vi "Setup UI.vi"(8 "error in (no error)":errorcluster, 10 "Set UI to input? (F)":bool, 11 "Two Lockins in":refnum<class "Two Lockins.lvclass">) -> (0 "error out":errorcluster, 3 "Two Lockins out":refnum<class "Two Lockins.lvclass">)   [LabVIEW 2023, in "Two Lockins.lvclass"]
doc: "Setup UI constructs an object -- populates its member fields -- from a front panel the user can see. The VI should be as simple as possible so that a UI loop can poll it continuously for updates. \n\nThe VI is designed to be used as a subPanel within another VI. Wire true to \"Set UI to input\" only on the first call, just after inserting this VI into a subPanel, to populate its controls with the class's current values.\n\nSetup UI is distinct from the class constructor. Class constructors are not polymorphic, yet configure dialogs need to configure objects without knowing their type -- and polymorphism is the necessary solution. Thus, Setup UI is a polymorphic class constructor. This continously polled \"Setup UI\" concept is a kludge: a better idea would be an XControl, but those require a steeper learning curve."
uses:
  Two Lockins.lvclass
  Lockin/Sensitivity.ctl
  Two Lockins.lvclass/Two Lockins.ctl
  Utility Classes/Readable/Readable.lvclass
  Lockin/sr830/SR830.lvlib
  Lockin/Lockin SR830.lvclass
panel:
  in  "Tau 2":u16(ring) items=["10 us", "30 us", "100 us", "300 us", "1 ms", "3 ms", "10 ms", "30 ms", "100 ms", "300 ms", "1 s", "3 s", "10 s", "30 s", "100 s", "300 s", "1 ks", "3 ks", "10 ks", "30 ks"]
  in  "Sensitivity 2":T1 items=["2 nV", "5 nV", "10 nV", "20 nV", "50 nV", "100 nV", "200 nV", "500 nV", "1 uV", "2 uV", "5 uV", "10 uV", "20 uV", "50 uV", "100 uV", "200 uV", "500 uV", "1 mV", "2 mV", "5 mV", "10 mV", "20 mV", "50 mV", "100 mV", "200 mV", "500 mV", "1 V"]
  in  "Reference mode 2":enum16{"external", "internal"}(ring)
  in  "Frequency 2":dbl[unit]
  in  "Set Parameters":bool
  in  "Tau":u16(ring) items=["10 us", "30 us", "100 us", "300 us", "1 ms", "3 ms", "10 ms", "30 ms", "100 ms", "300 ms", "1 s", "3 s", "10 s", "30 s", "100 s", "300 s", "1 ks", "3 ks", "10 ks", "30 ks"]
  in  "Sensitivity":T1 items=["2 nV", "5 nV", "10 nV", "20 nV", "50 nV", "100 nV", "200 nV", "500 nV", "1 uV", "2 uV", "5 uV", "10 uV", "20 uV", "50 uV", "100 uV", "200 uV", "500 uV", "1 mV", "2 mV", "5 mV", "10 mV", "20 mV", "50 mV", "100 mV", "200 mV", "500 mV", "1 V"]
  in  "Reference mode":enum16{"external", "internal"}(ring)
  in  "Frequency":dbl[unit]
  # "Two Lockins Instrument Setup"
  # "SR830"
  # "SR810"
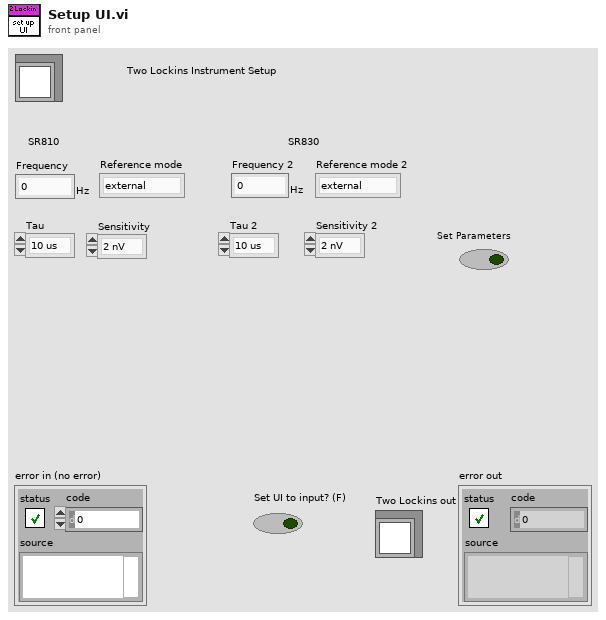
[diagram p1: front panel]
types:
  T1 = typedef "Lockin SR830.lvclass/Sensitivity.ctl" = u16
  T2 = typedef "SR830.lvlib/Tau.ctl" = u16
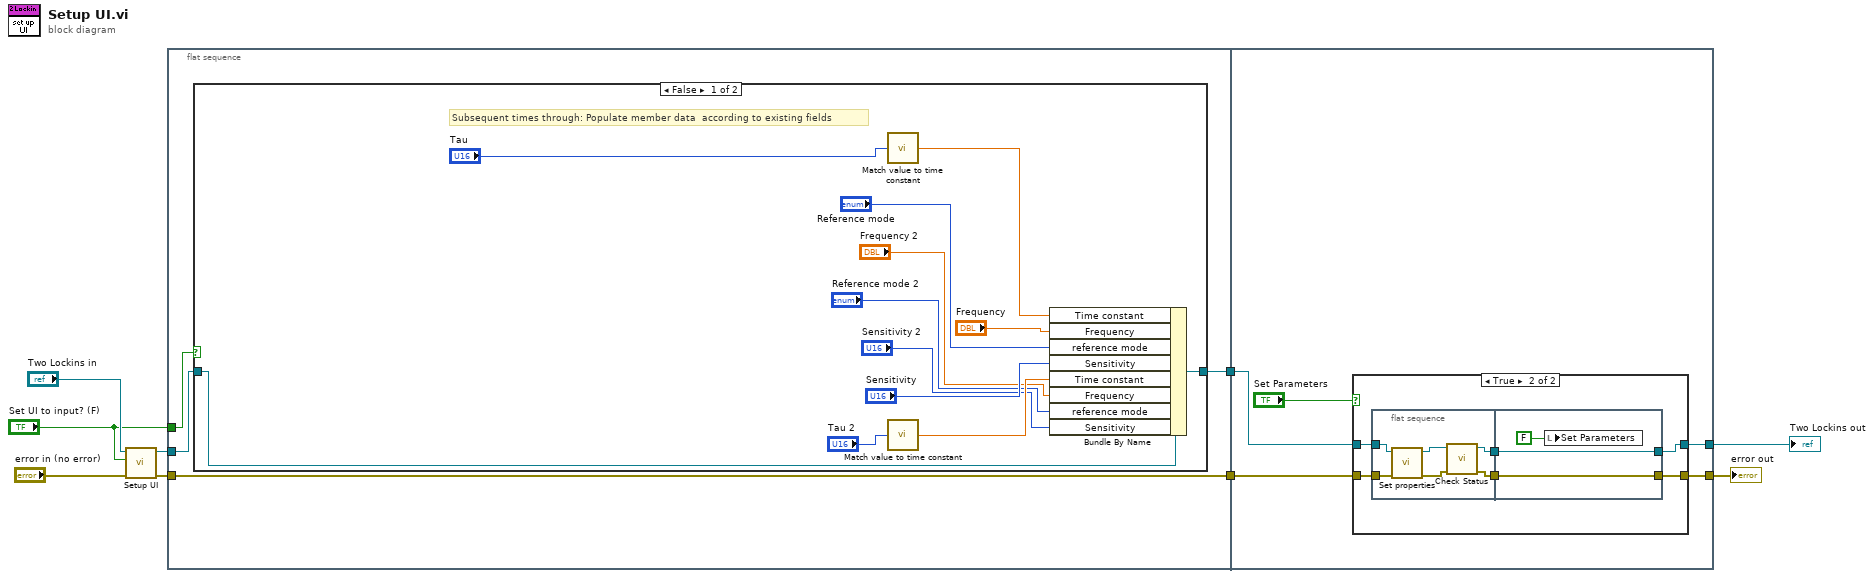
[diagram p0: block diagram]
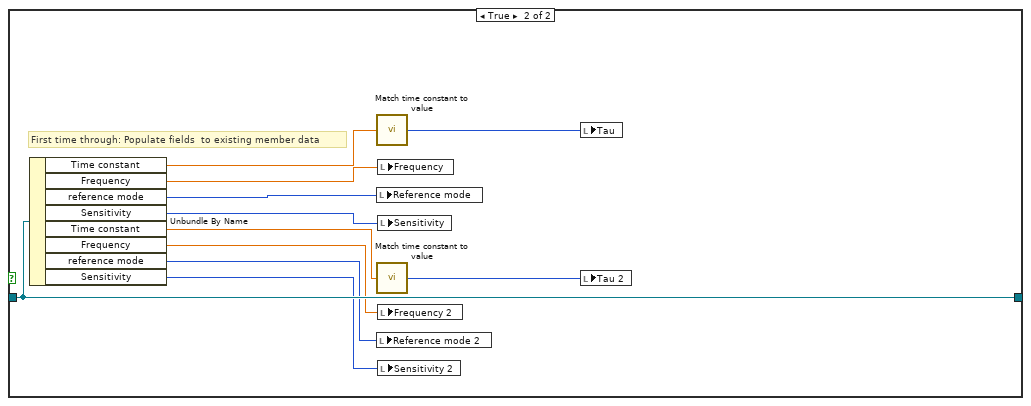
[diagram p2: hidden frame]
diagram:
  n1 = call-parent "Setup UI.vi"("error in (no error)"="error in (no error)", "Set UI to input? (F)"="Set UI to input? (F)", "Instrument in"="Two Lockins in") -> ("error out"=w4:errorcluster, "Instrument out"=w3:refnum<class "Two Lockins.lvclass">)  [unwired: 7 in]
  n2 = flat-sequence {
    tunnel: "Set UI to input? (F)" -> [w13]
    tunnel: w3 -> [w12]
    tunnel: [w11] -> w7
    tunnel: [w10] -> w6
    tunnel: w4 -> [w10]
    tunnel: w7 -> [w41]
    tunnel: [w38] -> w2
    tunnel: w6 -> [w40]
    tunnel: [w39] -> w1
    frame #0 {
      n3 = case shown="False" w13 {
        tunnel: w12 -> [w25 w35]
        tunnel: [w19 w35] -> w11
        frame False {
          # "Subsequent times through: Populate member data  according to existing fields"
          n4 = call "Match value to time constant.vi"("Tau"="Tau") -> ("time constant"=w24:dbl[unit])
          n5 = call "Match value to time constant.vi"("Tau"="Tau 2") -> ("time constant"=w17:dbl[unit])
          n6 = Bundle By Name(cluster=w25, "Time constant"=w24, "Frequency"="Frequency", "reference mode"="Reference mode", "Sensitivity"="Sensitivity", "Time constant"=w17, "Frequency"="Frequency 2", "reference mode"="Reference mode 2", "Sensitivity"="Sensitivity 2") -> (w19:refnum<class "Two Lockins.lvclass">)
        }
        frame True {
          # "First time through: Populate fields  to existing member data"
          n7 = Unbundle By Name(w35) -> ("Time constant"=w34:dbl[unit], "Frequency"=w33:dbl[unit], "reference mode"=w32:enum16{"external", "internal"}, "Sensitivity"=w31:T1, "Time constant"=w30:dbl[unit], "Frequency"=w28:dbl[unit], "reference mode"=w27:enum16{"external", "internal"}, "Sensitivity"=w26:T1)
          n8 = call "Match time constant to value.vi"("Time constant"=w34) -> ("Tau"=w36:T2)
          n9 = local write "Reference mode"(w32) -> ()
          n10 = call "Match time constant to value.vi"("Time constant"=w30) -> ("Tau"=w29:T2)
          n11 = local write "Reference mode 2"(w27) -> ()
          n12 = local write "Frequency"(w33) -> ()
          n13 = local write "Sensitivity"(w31) -> ()
          n14 = local write "Frequency 2"(w28) -> ()
          n15 = local write "Sensitivity 2"(w26) -> ()
          n16 = local write "Tau"(w36) -> ()
          n17 = local write "Tau 2"(w29) -> ()
        }
      }
    }
    frame #1 {
      n18 = case shown="True" "Set Parameters" {
        tunnel: w41 -> [w43 w49]
        tunnel: w40 -> [w42 w48]
        tunnel: [w42 w47] -> w39
        tunnel: [w43 w46] -> w38
        frame False {
        }
        frame True {
          n19 = flat-sequence {
            tunnel: w49 -> [w55]
            tunnel: w48 -> [w54]
            tunnel: [w50] -> w45
            tunnel: [w52] -> w44
            tunnel: [w57] -> w46
            tunnel: [w58] -> w47
            tunnel: w45 -> [w58]
            tunnel: w44 -> [w57]
            frame #0 {
              n20 = call "Set properties.vi"("error in (no error)"=w54, "Two Lockins in"=w55) -> ("error out"=w51:errorcluster, "Two Lockins out"=w53:refnum<class "Two Lockins.lvclass">)  [unwired: 8 in]
              n21 = call-dynamic "Check Status.vi"("error in (no error)"=w51, "Two Lockins in"=w53) -> ("error out"=w50:errorcluster, "Two Lockins out"=w52:refnum<class "Two Lockins.lvclass">)  [unwired: 6 in, 2 out]
            }
            frame #1 {
              n22 = local write "Set Parameters"(FALSE) -> ()
            }
          }
        }
      }
    }
  }
  "error out" <- w1
  "Two Lockins out" <- w2
